vi "VD-get_command.vi"(7 "Write?":bool, 10 "action":T3=enum."SweepStartHz") -> (2 "Command":T2 format="%x")   [LabVIEW 2020, in "VD-LV-LiteVNA.lvclass"]
uses:
  VD-LV-LiteVNA.lvclass
  VD-action.ctl
  hardware-protocol/serial/HP-S-data.ctl
  VD-command.ctl
  hardware-protocol/serial/HP-S-Serial.lvclass
panel:
  out "command":T1
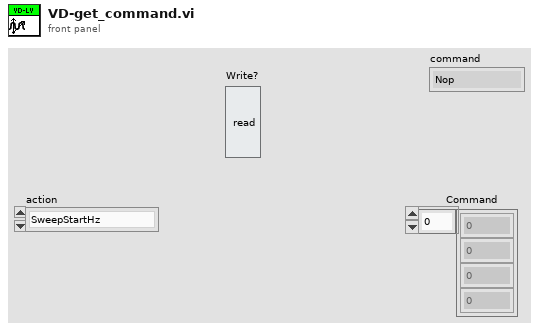
[diagram p1: front panel]
types:
  T1 = typedef "VD-LV-LiteVNA.lvclass/VD-command.ctl" = enum16{"Nop", "Indicate", "Read 1B", "Read 2B", "Read 4B", "Read 8B", "Read FIFO", "Write 1B", "Write 2B", "Write 4B", "Write 8B", "Write FIFO"}
  T2 = typedef "HP-S-Serial.lvclass/HP-S-data.ctl" = u8[]
  T3 = typedef "VD-LV-LiteVNA.lvclass/VD-action.ctl" = enum16{"checkCom", "SweepStartHz", "SweepStopHz", "SweepPoints", "valuesPerFrequency", "RawSamplesMode", "ValuesFIFO", "deviceVariant", "protocolVersion", "hardwareRevision", "firmwareMajor", "firmwareMinor"}
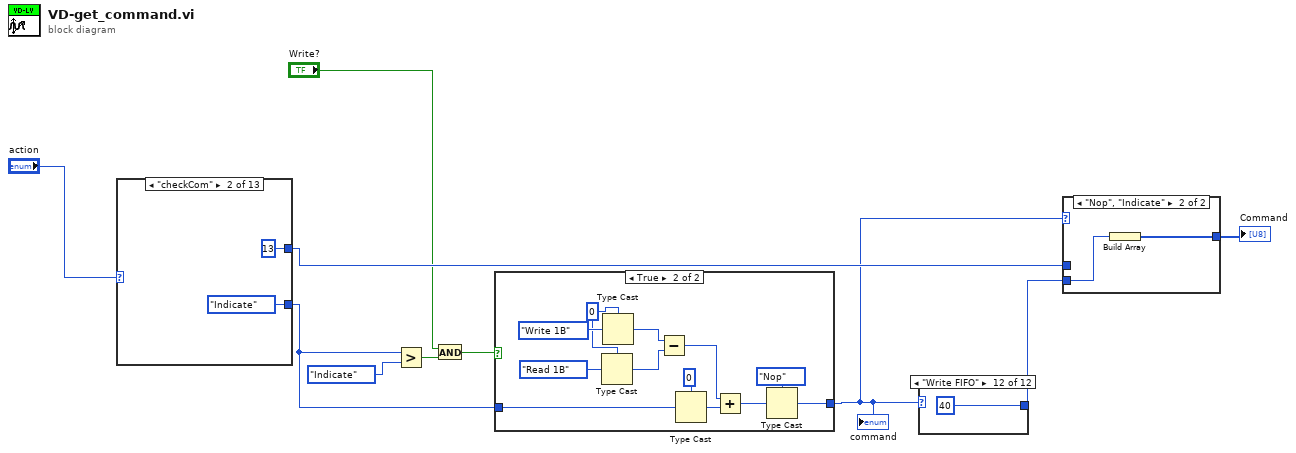
[diagram p0: block diagram]
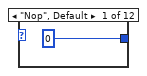
[diagram p3: hidden frame]
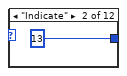
[diagram p4: hidden frame]
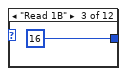
[diagram p5: hidden frame]
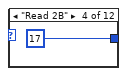
[diagram p6: hidden frame]
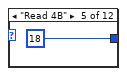
[diagram p7: hidden frame]
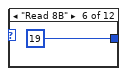
[diagram p8: hidden frame]
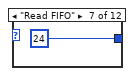
[diagram p9: hidden frame]
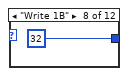
[diagram p10: hidden frame]
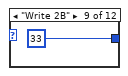
[diagram p11: hidden frame]
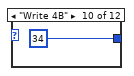
[diagram p12: hidden frame]
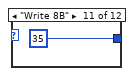
[diagram p13: hidden frame]
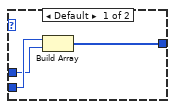
[diagram p14: hidden frame]
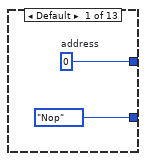
[diagram p15: hidden frame]
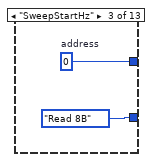
[diagram p16: hidden frame]
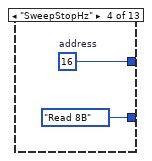
[diagram p17: hidden frame]
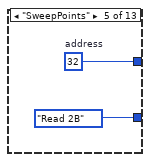
[diagram p18: hidden frame]
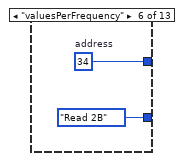
[diagram p19: hidden frame]
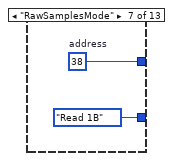
[diagram p20: hidden frame]
diagram:
  n1 = case shown="\"checkCom\"" "action" {
    tunnel: [w12 u8 13 ("address") w16 w18 w20 w22 w24 w26 w28 w30 w32 w34 w36] -> w10
    tunnel: [VD-command."Nop" ("command") VD-command."Indicate" ("command") VD-command."Read 8B" ("command") VD-command."Read 8B" ("command") VD-command."Read 2B" ("command") VD-command."Read 2B" ("command") VD-command."Read 1B" ("command") VD-command."Read FIFO" ("command") VD-command."Read 1B" ("command") VD-command."Read 1B" ("command") VD-command."Read 1B" ("command") VD-command."Read 1B" ("command") VD-command."Read 1B" ("command")] -> w5
    frame Default {
      w12 = u8 0  # address
    }
    frame "checkCom" {
    }
    frame "SweepStartHz" {
      w16 = u8 0  # address
    }
    frame "SweepStopHz" {
      w18 = u8 16  # address
    }
    frame "SweepPoints" {
      w20 = u8 32  # address
    }
    frame "valuesPerFrequency" {
      w22 = u8 34  # address
    }
    frame "RawSamplesMode" {
      w24 = u8 38  # address
    }
    frame "ValuesFIFO" {
      w26 = u8 48  # address
    }
    frame "deviceVariant" {
      w28 = u8 240  # address
    }
    frame "protocolVersion" {
      w30 = u8 241  # address
    }
    frame "hardwareRevision" {
      w32 = u8 242  # address
    }
    frame "firmwareMajor" {
      w34 = u8 243  # address
    }
    frame "firmwareMinor" {
      w36 = u8 244  # address
    }
  }
  n2 = Greater?(x=w5, y=VD-command."Indicate" ("command")) -> (0:w4:bool)
  n3 = And(x="Write?", y=w4) -> (x .and. y?=w3:bool)
  n4 = case shown="True" w3 {
    tunnel: w5 -> [w37 w42]
    tunnel: [w37 w38] -> w1
    frame False {
    }
    frame True {
      w48 = u16 0
      n5 = Type Cast(type=w48, x=VD-command."Read 1B" ("command")) -> (*(type *) &x=w45:u16)
      n6 = Type Cast(type=w48, x=VD-command."Write 1B" ("command")) -> (*(type *) &x=w46:u16)
      n7 = Subtract(x=w46, y=w45) -> (x-y=w41:u16)
      n8 = Type Cast(type=u16 0, x=w42) -> (*(type *) &x=w43:u16)
      n9 = Add(x=w41, y=w43) -> (x+y=w40:u16)
      n10 = Type Cast(type=VD-command."Nop" ("command"), x=w40) -> (*(type *) &x=w38:T1)
    }
  }
  "command" <- w1
  n11 = case shown="\"Write FIFO\"" w1 {
    tunnel: [u8 0 u8 13 u8 16 u8 17 u8 18 u8 19 u8 24 u8 32 u8 33 u8 34 u8 35 u8 40] -> w9
    frame "Nop", Default {
    }
    frame "Indicate" {
    }
    frame "Read 1B" {
    }
    frame "Read 2B" {
    }
    frame "Read 4B" {
    }
    frame "Read 8B" {
    }
    frame "Read FIFO" {
    }
    frame "Write 1B" {
    }
    frame "Write 2B" {
    }
    frame "Write 4B" {
    }
    frame "Write 8B" {
    }
    frame "Write FIFO" {
    }
  }
  n12 = case shown="\"Nop\", \"Indicate\"" w1 {
    tunnel: w10 -> [w63 _]
    tunnel: w9 -> [w64 w66]
    tunnel: [w62 w65] -> w2
    frame Default {
      n13 = Build Array(w64, w63) -> (w62:u8[])
    }
    frame "Nop", "Indicate" {
      n14 = Build Array(w66) -> (w65:u8[])
    }
  }
  "Command" <- w2
